vi "UpdateChannel.vi"(8 "error in":errorcluster, 10 "UpdatedChannel.lvclass":refnum<class "T560Channel.lvclass">, 11 "T560Session in":refnum<class "T560Session.lvclass">) -> (0 "error out":errorcluster, 3 "T560Session out":refnum<class "T560Session.lvclass">)   [LabVIEW 2013, in "T560Session.lvclass"]
doc: "Update the specified channel properties"
uses:
  T560Session.lvclass
  T560ChannelClass/T560Channel.lvclass
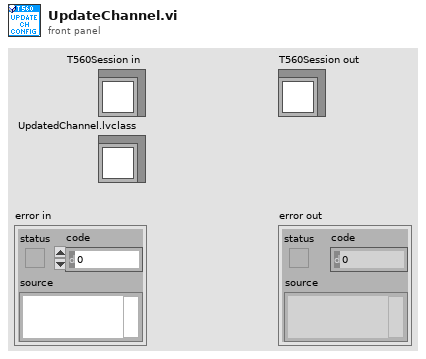
[diagram p1: front panel]
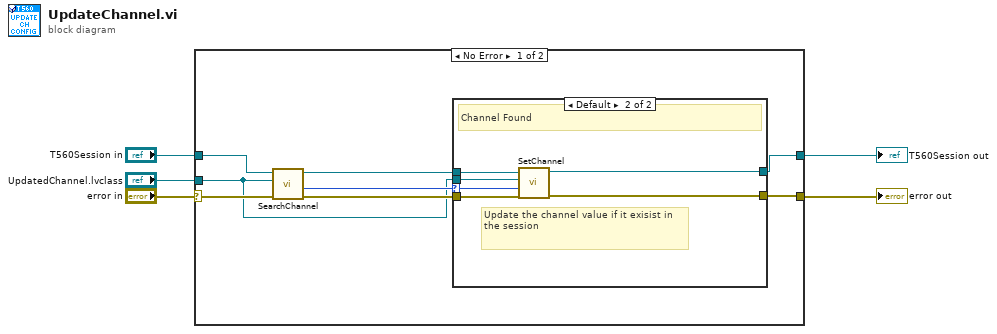
[diagram p0: block diagram]
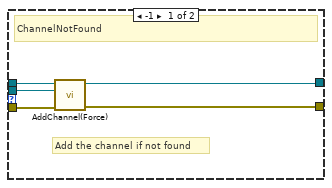
[diagram p2: hidden frame]
diagram:
  n1 = case shown="No Error" "error in" {
    selector: "error in" -> [w8 w26]
    tunnel: [w11 w26] -> w4
    tunnel: [w9 w25] -> w1
    tunnel: "T560Session in" -> [w13 w25]
    tunnel: "UpdatedChannel.lvclass" -> [w6 _]
    frame No Error {
      n2 = call-dynamic "SearchChannel.vi"("error in"=w8, "T560Channel.lvclass"=w6, "T560Session in"=w13) -> ("error out"=w12:errorcluster, "Index"=w7:i32, "T560Session out"=w10:refnum<class "T560Session.lvclass">)  [unwired: 5 in, 1 out]
      n3 = case shown="Default" w7 {
        selector: w7 -> [_ w19]
        tunnel: w12 -> [w18 w24]
        tunnel: [w15 w23] -> w11
        tunnel: w10 -> [w14 w22]
        tunnel: [w16 w21] -> w9
        tunnel: w6 -> [w17 w20]
        frame -1 {
          # "Add the channel if not found"
          # "ChannelNotFound"
          n4 = call-dynamic "AddChannel(Force).vi"("error in (no error)"=w18, "T560Channel.lvclass"=w17, "T560Session in"=w14) -> ("error out"=w15:errorcluster, "T560Session out"=w16:refnum<class "T560Session.lvclass">)  [unwired: 7 in]
        }
        frame Default {
          # "Update the channel value if it exisist in the session"
          # "Channel Found"
          n5 = call-dynamic "SetChannel.vi"("error in"=w24, "index"=w19, "T560Channel.lvclass"=w20, "T560Session in"=w22) -> ("error out"=w23:errorcluster, "T560Session out"=w21:refnum<class "T560Session.lvclass">)  [unwired: 6 in]
        }
      }
    }
    frame Error {
    }
  }
  "error out" <- w4
  "T560Session out" <- w1
